vi "Configure DigitalIn.vi"(10 "Samplerate In":T1=8192 min=10 max=100000000 step=10, 11 "ADALM2000 Handler":u32 caption="Instrument Handle Out") -> (3 "ADALM2000 Handler 2":u32 caption="Instrument Handle Out")   [LabVIEW 2015]
uses:
  Controls/SampleRateControlDig.ctl
  libm2k_lv.dll
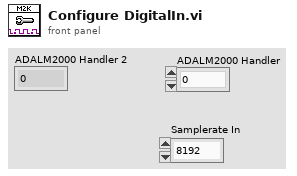
[diagram p1: front panel]
types:
  T1 = typedef "SampleRateControlDig.ctl" = i32
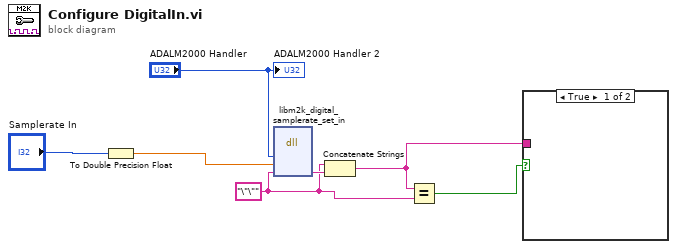
[diagram p0: block diagram]
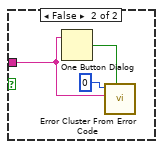
[diagram p2: hidden frame]
diagram:
  w4 = "\"\""
  n1 = To Double Precision Float(number="Samplerate In") -> (double precision float=w7:dbl)
  n2 = dll-call lib="libm2k_lv.*" fn="libm2k_digital_samplerate_set_in"("instance"="ADALM2000 Handler", "samplerate"=w7, "err"=w4) -> ("err"=w6:string)  [unwired: 6 in, 2 out]
  n3 = Concatenate Strings(w4, w6) -> (w2:string)
  n4 = Equal?(x=w2, y=w4) -> (x = y?=w3:bool)
  n5 = case shown="True" w3 {
    tunnel: w2 -> [_ w8]
    frame True {
    }
    frame False {
      n6 = One Button Dialog(message=w8) -> (true=w10:bool)  [unwired: 1 in]
      n7 = call <vilib>:"Error Cluster From Error Code.vi"("show call chain? (False)"=w10, "error message (\"\")"=w8, "error code (0)"=0) -> ()  [unwired: 6 in, 1 out]
    }
  }
  "ADALM2000 Handler 2" <- "ADALM2000 Handler"
